vi "Configure Bus Source (SPI - Idle Time).vi"(0 "VISA resource name":refnum<visa-resource-name>, 1 "MOSI":T3={"MOSI Source (30: Off)"=30, "MOSI Polarity (0: High)"=0} {"MOSI Polarity (0: High)" items=["Active High", "Active Low"]; "MOSI Source (30: Off)" items=["Channel 1"=0, "Channel 2"=1, "Channel 3"=2, "Channel 4"=3, "Digital Channel 0"=14, "Digital Channel 1"=15, "Digital Channel 2"=16, "Digital Channel 3"=17, "Digital Channel 4"=18, "Digital Channel 5"=19, "Digital Channel 6"=20, "Digital Channel 7"=21, "Digital Channel 8"=22, "Digital Channel 9"=23, "Digital Channel 10"=24, "Digital Channel 11"=25, "Digital Channel 12"=26, "Digital Channel 13"=27, "Digital Channel 14"=28, "Digital Channel 15"=29, "Off"=30]}, 2 "MISO":T2={"MISO Source (30: Off)"=30, "MISO Polarity (0: High)"=0} {"MISO Polarity (0: High)" items=["Active High", "Active Low"]; "MISO Source (30: Off)" items=["Channel 1"=0, "Channel 2"=1, "Channel 3"=2, "Channel 4"=3, "Digital Channel 0"=14, "Digital Channel 1"=15, "Digital Channel 2"=16, "Digital Channel 3"=17, "Digital Channel 4"=18, "Digital Channel 5"=19, "Digital Channel 6"=20, "Digital Channel 7"=21, "Digital Channel 8"=22, "Digital Channel 9"=23, "Digital Channel 10"=24, "Digital Channel 11"=25, "Digital Channel 12"=26, "Digital Channel 13"=27, "Digital Channel 14"=28, "Digital Channel 15"=29, "Off"=30]}, 5 "BUS Number (9: Bus 1)":u16(ring)=9 items=["Bus 1"=9, "Bus 2"=10, "Bus 3"=11, "Bus 4"=12], 7 "SCLK":T1 {"SCLK Polarity (0: Rising)" items=["Rising", "Falling"]; "SCLK Source (0: Channel 1)" items=["Channel 1"=0, "Channel 2"=1, "Channel 3"=2, "Channel 4"=3, "Digital Channel 0"=14, "Digital Channel 1"=15, "Digital Channel 2"=16, "Digital Channel 3"=17, "Digital Channel 4"=18, "Digital Channel 5"=19, "Digital Channel 6"=20, "Digital Channel 7"=21, "Digital Channel 8"=22, "Digital Channel 9"=23, "Digital Channel 10"=24, "Digital Channel 11"=25, "Digital Channel 12"=26, "Digital Channel 13"=27, "Digital Channel 14"=28, "Digital Channel 15"=29]}, 9 "Idle Time (100 ns)":dbl=1e-07 format="%^#_6g", 11 "error in (no error)":errorcluster, 12 "Word Size (8 Bits)":u8=8, 13 "Bit Order (0: Most Significant First)":u16(ring) items=["Most Significant First", "Least Significant First"]) -> (4 "VISA resource name out":refnum<visa-resource-name>, 15 "error out":errorcluster)   [LabVIEW 2009, in "Tektronix DPO MSO 2000 4000 Series.lvlib"]
doc: "Configures SPI bus with Idle Time framing (non-standard 2 wire) settings for an oscilloscope.\n\n<B>Note:</B>\n\nFor SS framing (standard 3-wire SPI), use <B>Configure Bus Source (SPI)</B> VI instead."
uses:
  <instrlib>/Tektronix DPO MSO 2000 4000 Series/Tektronix DPO MSO 2000 4000 Series.lvlib
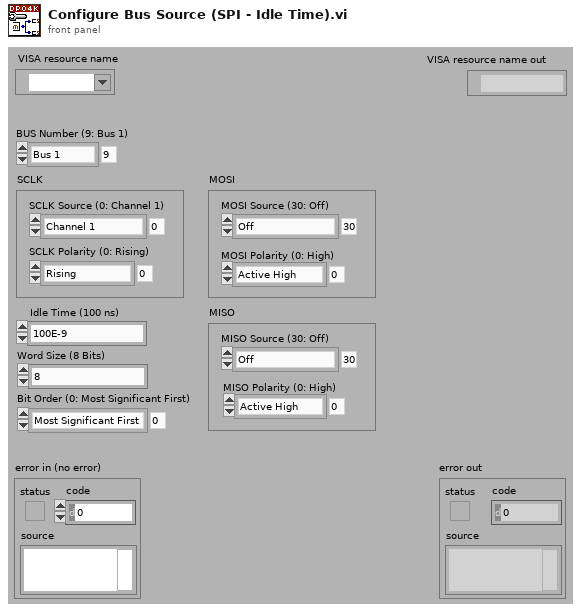
[diagram p1: front panel]
types:
  T1 = cluster{"SCLK Source (0: Channel 1)":u16, "SCLK Polarity (0: Rising)":u16}
  T2 = cluster{"MISO Source (30: Off)":u16, "MISO Polarity (0: High)":u16}
  T3 = cluster{"MOSI Source (30: Off)":u16, "MOSI Polarity (0: High)":u16}
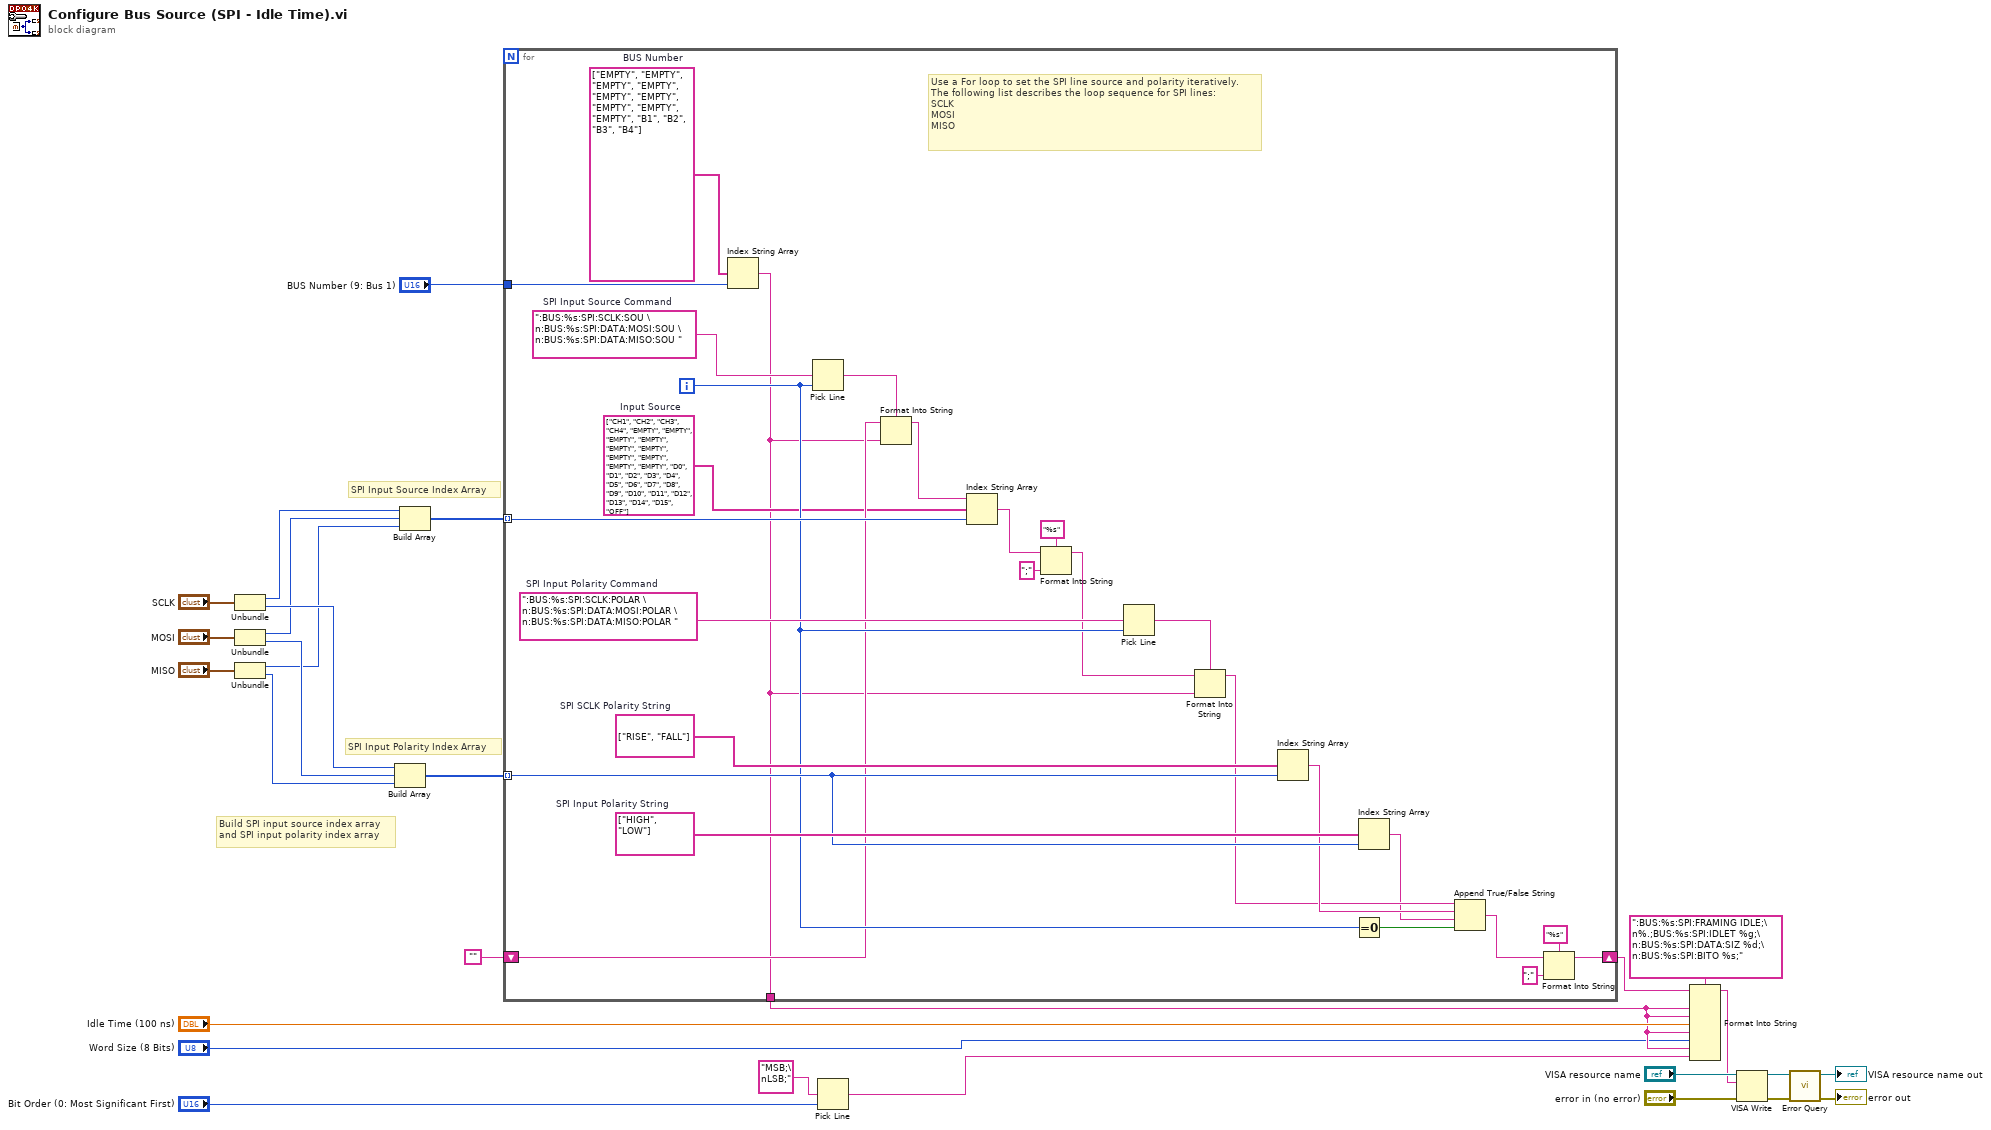
[diagram p0: block diagram]
diagram:
  # "Build SPI input source index array\nand SPI input polarity index array"
  # "SPI Input Polarity Index Array"
  # "SPI Input Source Index Array"
  n1 = Unbundle("SCLK") -> ("SCLK Source (0: Channel 1)"=w25:u16, "SCLK Polarity (0: Rising)"=w24:u16)
  n2 = Unbundle("MOSI") -> ("MOSI Source (30: Off)"=w8:u16, "MOSI Polarity (0: High)"=w10:u16)
  n3 = Unbundle("MISO") -> ("MISO Source (30: Off)"=w7:u16, "MISO Polarity (0: High)"=w9:u16)
  n4 = Build Array(w24, w10, w9) -> (w22:u16[])
  n5 = Build Array(w25, w8, w7) -> (w23:u16[])
  n6 = for {
    tunnel: w23 -> [w52] mode=indexing
    tunnel: w22 -> [w46] mode=indexing
    shift-right: [w36] -> w13
    shift-left: "" -> [w33]
    tunnel: "BUS Number (9: Bus 1)" -> [w30]
    tunnel: [w29] -> w2
    i -> [w43]
    w32 = string[] ["CH1", "CH2", "CH3", "CH4", "EMPTY", "EMPTY", "EMPTY", "EMPTY", "EMPTY", "EMPTY", "EMPTY", "EMPTY", "EMPTY", "EMPTY", "D0", "D1", "D2", "D3", "D4", "D5", "D6", "D7", "D8", "D9", "D10", "D11", "D12", "D13", "D14", "D15", "OFF"]  # Input Source
    w53 = string[] ["EMPTY", "EMPTY", "EMPTY", "EMPTY", "EMPTY", "EMPTY", "EMPTY", "EMPTY", "EMPTY", "B1", "B2", "B3", "B4"]  # BUS Number
    w51 = string[] ["RISE", "FALL"]  # SPI SCLK Polarity String
    w47 = string[] ["HIGH", "LOW"]  # SPI Input Polarity String
    w54 = ":BUS:%s:SPI:SCLK:POLAR \n:BUS:%s:SPI:DATA:MOSI:POLAR \n:BUS:%s:SPI:DATA:MISO:POLAR "  # SPI Input Polarity Command
    w55 = ":BUS:%s:SPI:SCLK:SOU \n:BUS:%s:SPI:DATA:MOSI:SOU \n:BUS:%s:SPI:DATA:MISO:SOU "  # SPI Input Source Command
    # "Use a For loop to set the SPI line source and polarity iteratively.\nThe following list describes the loop sequence for SPI lines:\nSCLK\nMOSI\nMISO"
    n7 = Index String Array(1:w30, 2:w53) -> (0:w29:string)  [unwired: 1 in]
    n8 = Pick Line(multi-line string=w55, line index=w43) -> (output string=w37:string)  [unwired: 1 in]
    n9 = Format Into String(format string=w37, initial string=w33, w29) -> (resulting string=w45:string)  [unwired: 1 in, 1 out]
    n10 = Index String Array(1:w52, 2:w32, 3:w45) -> (0:w50:string)
    n11 = Format Into String(format string="%s", initial string=w50, ";" ("input 1")) -> (resulting string=w31:string)  [unwired: 1 in, 1 out]
    n12 = Pick Line(multi-line string=w54, line index=w43) -> (output string=w44:string)  [unwired: 1 in]
    n13 = Format Into String(format string=w44, initial string=w31, w29) -> (resulting string=w40:string)  [unwired: 1 in, 1 out]
    n14 = Index String Array(1:w46, 2:w51) -> (0:w41:string)  [unwired: 1 in]
    n15 = Equal To 0?(x=w43) -> (x = 0?=w42:bool)
    n16 = Index String Array(1:w46, 2:w47) -> (0:w35:string)  [unwired: 1 in]
    n17 = Append True/False String(1:w42, 2:w35, 3:w41, 4:w40) -> (0:w34:string)
    n18 = Format Into String(format string="%s", initial string=w34, ";" ("input 1")) -> (resulting string=w36:string)  [unwired: 1 in, 1 out]
  }
  n19 = Pick Line(multi-line string="MSB;\nLSB;", line index="Bit Order (0: Most Significant First)") -> (output string=w3:string)  [unwired: 1 in]
  n20 = Format Into String(format string=":BUS:%s:SPI:FRAMING IDLE;\n%.;BUS:%s:SPI:IDLET %g;\n:BUS:%s:SPI:DATA:SIZ %d;\n:BUS:%s:SPI:BITO %s;" ("input 1"), initial string=w13, w2, w2, "Idle Time (100 ns)", w2, "Word Size (8 Bits)", w2, w3) -> (resulting string=w12:string)  [unwired: 1 in, 1 out]
  n21 = VISA Write(VISA resource name="VISA resource name", write buffer=w12, error in (no error)="error in (no error)") -> (VISA resource name out=w20:refnum<visa-resource-name>, error out=w19:errorcluster)  [unwired: 1 out]
  n22 = call <instrlib>:"Error Query.vi"("error in (no error)"=w19, "VISA resource name"=w20) -> ("error out"=→"error out":errorcluster, "VISA resource name out"=→"VISA resource name out":refnum<visa-resource-name>)  [unwired: 6 in, 2 out]
